vi "Delete from Array (Multi).vi"(8 "index":i32, 9 "length":i32, 11 "JSON Array In":refnum<class "JSON Value.lvclass">) -> (1 "deleted portion":refnum<class "JSON Value.lvclass">[](array[class]), 3 "JSON Array w/ subset deleted":refnum<class "JSON Value.lvclass">)   [LabVIEW 2016, in "JSON Value.lvclass"]
doc: "Deletes an element or subarray from a JSON array of length elements starting at index. Returns the edited array in array w/ subset deleted and the deleted element or subarray in deleted portion."
uses:
  JSON Value.lvclass
  JSON Value.lvclass/JSON Value.ctl
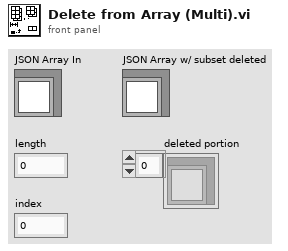
[diagram p1: front panel]
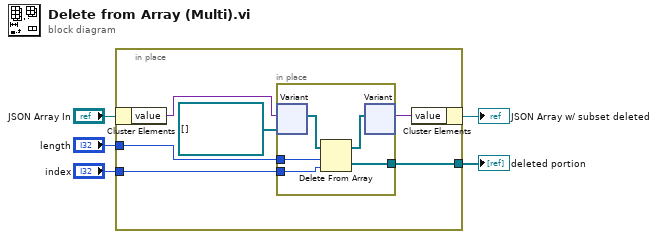
[diagram p0: block diagram]
diagram:
  n1 = in-place {
    in-place-border: "index" -> [w11]
    in-place-border: [w10] -> w1
    in-place-border: "length" -> [w9]
    n2 = in-place-cluster #1("JSON Array In") -> ("value"=w7:variant)
    n3 = in-place {
      in-place-border: w11 -> [w16]
      in-place-border: [w15] -> w10
      in-place-border: w9 -> [w14]
      n4 = in-place-variant #2(w7, refnum<class "JSON Value.lvclass">[] [] ("JSON Array In")) -> (w13:refnum<class "JSON Value.lvclass">[])  [unwired: 1 out]
      n5 = Delete From Array(array=w13, length=w14, index=w16) -> (deleted portion=w15:refnum<class "JSON Value.lvclass">[], array with subset deleted=w12:refnum<class "JSON Value.lvclass">[])
      n6 = in-place-variant #2(w12) -> (w6:variant)  [unwired: 1 out]
    }
    n7 = in-place-cluster #1("value"=w6) -> (→"JSON Array w/ subset deleted":refnum<class "JSON Value.lvclass">)
  }
  "deleted portion" <- w1
